vi "niUSRP EX Full Duplex (Single Device, Multi Channel)-20221205.vi"() -> ()   [LabVIEW 2021]
doc: "Continuously acquires and generates two communications signals in a synchronous manner using both channels on a two channel device."
uses:
  <instrlib>/niUSRP/niUSRP Timestamp.ctl
  <vilib>/Analysis/3filter.llb/Filter Passband Type.ctl
  <instrlib>/niUSRP/niUSRP Configure Time Start Trigger.vi
  <vilib>/Analysis/3filter.llb/Butterworth Filter (CDB).vi
  <instrlib>/niUSRP/niUSRP Fetch Rx Data (2D CDB).vi
  <vilib>/measure/maspectr.llb/FFT Power Spectrum for 1 Chan (CDB).vi
  <instrlib>/niUSRP/niUSRP Write Tx Data (2D CDB).vi
  <vilib>/measure/NI_MABase.lvlib
  <vilib>/measure/NI_MAPro.lvlib
  <vilib>/Analysis/NI_AALBase.lvlib
panel:
  out "error":i32
  in  "filter type":T1=enum."Bandpass"
  out "appended array":cdb[][](array[numeric])
  in  "low cutoff freq: fl":dbl=0.12500000000000006 format="%^.4e"
  in  "high cutoff freq: fh":dbl=0.45000000000000007 format="%^.2e"
  in  "sampling freq: fs":dbl=1.0 format="%^.2e"
  out "IQ Graph 2":dbl[][](graph)
  out "Model":string
  out "error out":errorcluster
  in  "Tab Control 2":enum32{"NI-294x/295x/X410", "NI-2900/2901"}(tab)
  in  "channel 0 carrier\n frequency [Hz]":dbl=2000000000.0 format="%#_6p"
  in  "channel 1 carrier\n frequency [Hz]":dbl=2000000000.0 format="%#_6p"
  in  "Start Trigger Time":T2={"whole seconds"=1, "fractional seconds"=0.0}
  in  "Tx Active Antenna":string="TX1"
  in  "Tab Control":T3(tab)
  out "IQ Graph":dbl[][](graph)
  out "Baseband Power Spectrum":cluster{"f0":dbl, "df":dbl, "magnitude":dbl[]}[](graph)
  in  "Stop":bool
  in  "Channel 1\nTone Amplitude":dbl=0.4 step=0.05 format="%#.6g"
  in  "Channel 1\nTone Frequency":dbl=35000.0 format="%#_6p"
  in  "Channel 0\nTone Amplitude":dbl=0.707 step=0.05 format="%#.6g"
  in  "Channel 0 \nTone Frequency":dbl=10000.0 format="%#_6p"
  out "Tx Waveform Graph":waveform(dbl)[](graph)
  in  "Waveform Size":dbl=10000.0
  in  "Rx Active Antenna":string="RX2"
  in  "Device Name":refnum<k15>="X310"
  in  "Tx Gain":dbl=1.0 format="%#_6f"
  in  "Tx IQ Rate":dbl=1000000.0 format="%#_6p"
  in  "Rx Gain":dbl=1.0 format="%#_6f"
  in  "Rx IQ Rate":dbl=1000000.0 format="%#_6p"
  # "Rx Settings"
  # "Tx Settings"
  # "For X410 use TX/RX0"
  # "Note that on the NI-2900 and NI-2901, both Rx channels share an LO and both Tx channels share an LO. However, on the NI-294x/295x devices, Rx and Tx of channel 0 share an LO and Rx and Tx of channel 1 share an LO."
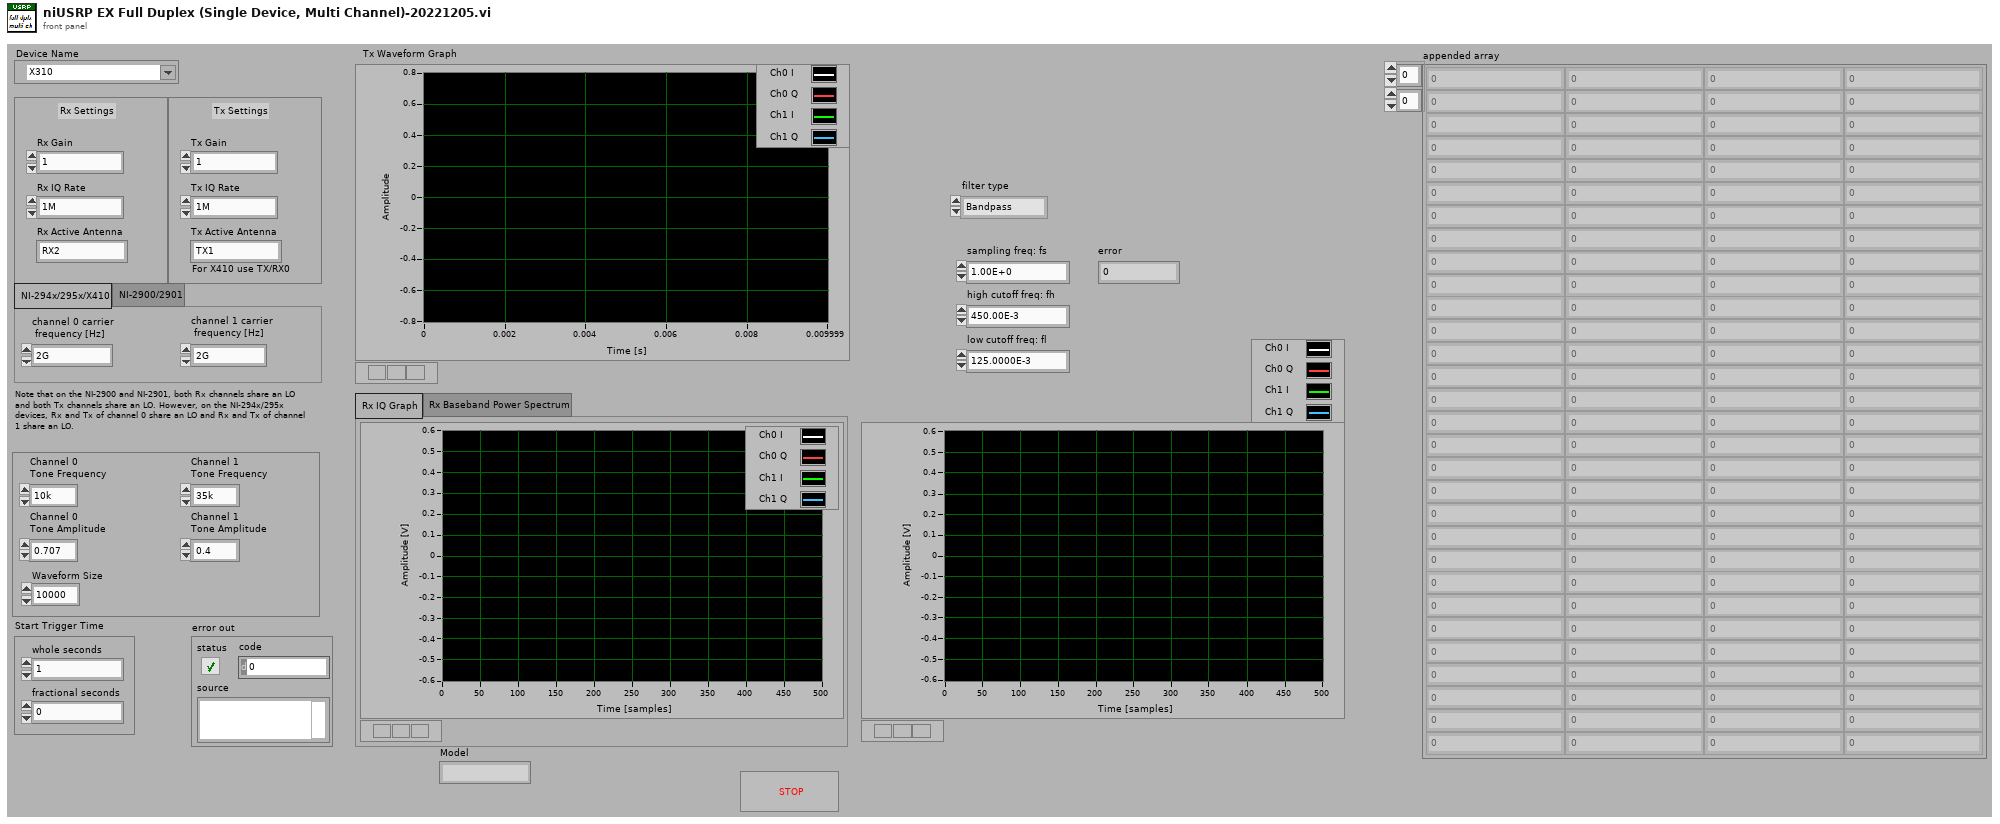
[diagram p1: front panel]
types:
  T1 = typedef "NI_AALBase.lvlib/Filter Passband Type.ctl" = enum32{"Lowpass", "Highpass", "Bandpass", "Bandstop"}
  T2 = typedef "niUSRP Timestamp.ctl" = cluster{"whole seconds":u64, "fractional seconds":dbl}
  T3 = enum32{"Rx IQ Graph", "Rx Baseband Power Spectrum"}
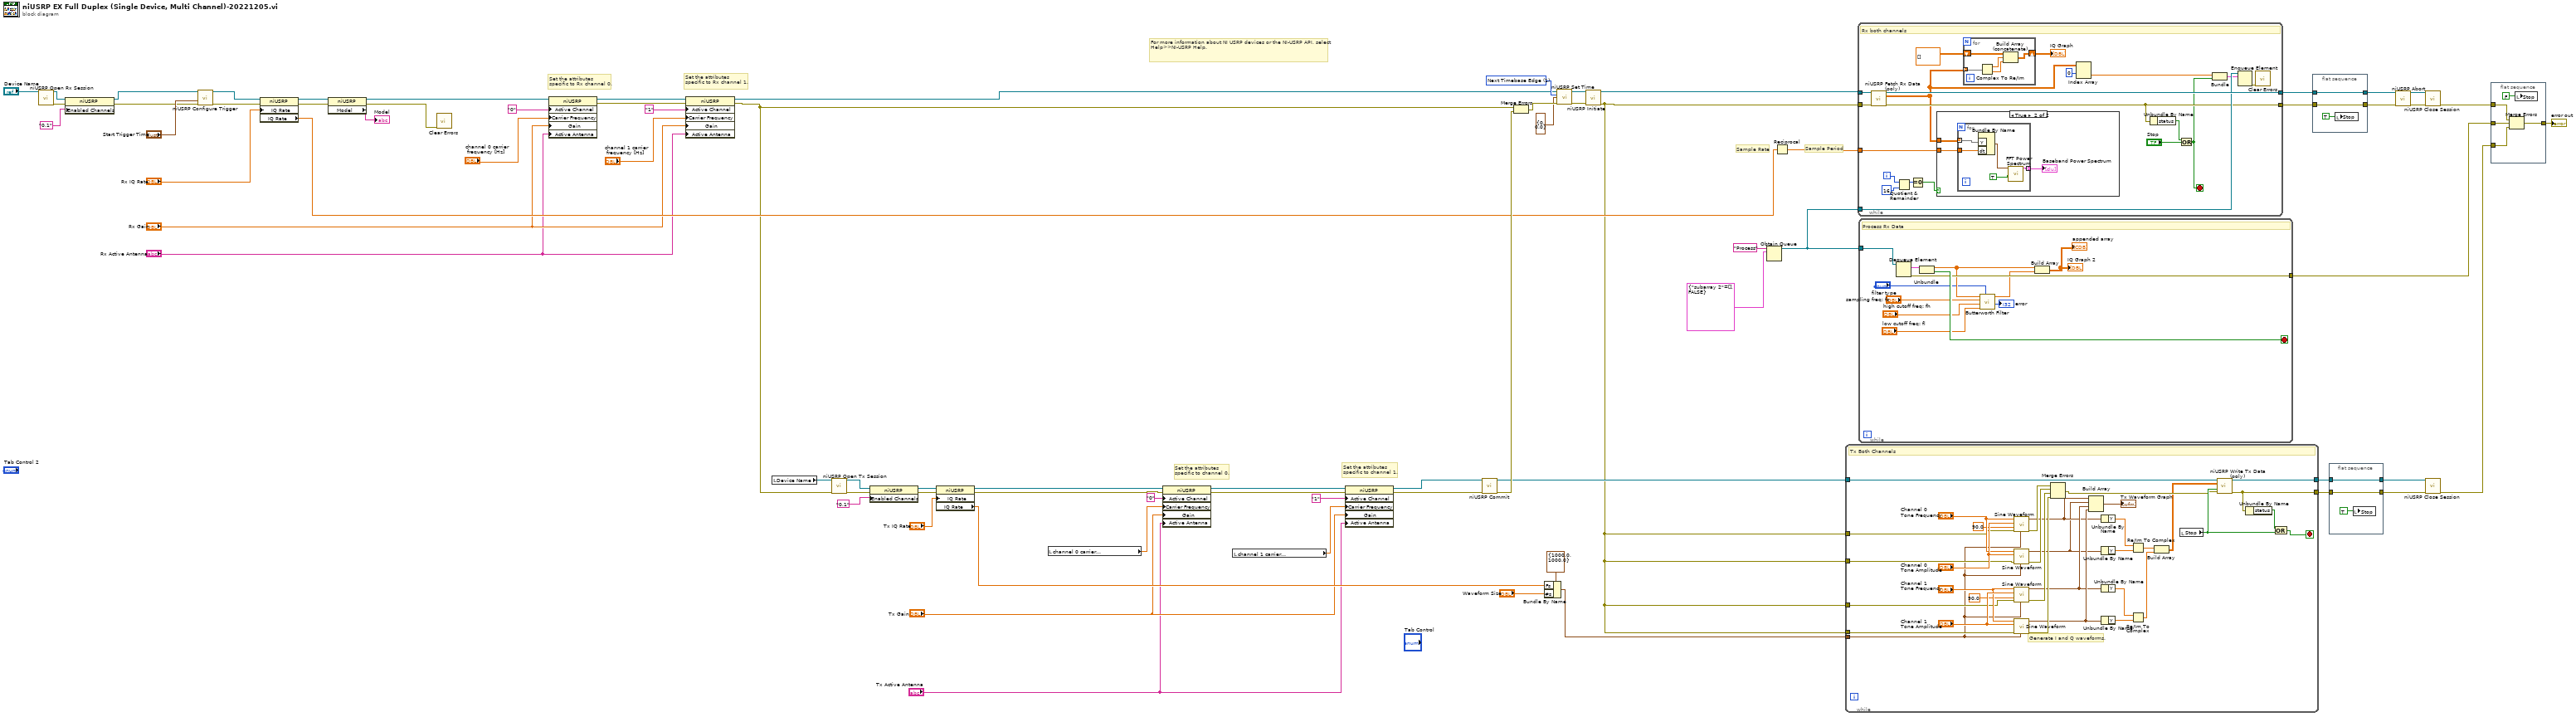
[diagram p0: block diagram]
diagram:
  w59 = 1 items=["Now", "Next Timebase Edge"] ("apply timestamp")
  # "Set the attributes \nspecific to channel 1."
  # "Set the attributes \nspecific to channel 0."
  # "Set the attributes \nspecific to Rx channel 1."
  # "Set the attributes \nspecific to Rx channel 0."
  # "Sample Rate"
  # "Sample Period"
  # "For more information about NI USRP devices or the NI-USRP API, select Help>>NI-USRP Help."
  n1 = call <instrlib>:"niUSRP Open Rx Session.vi"("device names"="Device Name") -> ("session handle out"=w58:refnum<k15>, "error out"=w57:errorcluster)  [unwired: 13 in]
  n2 = property class="niUSRP"(reference=w58, error in=w57, "Enabled Channels"="0,1" ("Configuration:Enabled Channels")) -> (reference out=w56:refnum<k15>, error out=w55:errorcluster)
  n3 = call-poly <instrlib>:"niUSRP Configure Trigger.vi"("session handle"=w56, "start trigger time"="Start Trigger Time", "error in (no error)"=w55) -> ("session handle out"=w52:refnum<k15>, "error out"=w51:errorcluster)  [unwired: 11 in]
  n4 = property class="niUSRP"(reference=w52, error in=w51, "IQ Rate"="Rx IQ Rate") -> (reference out=w47:refnum<k15>, error out=w48:errorcluster, "IQ Rate"=w49:dbl)
  n5 = property class="niUSRP"(reference=w47, error in=w48) -> (reference out=w44:refnum<k15>, error out=w5:errorcluster, "Model"=→"Model":string)
  n6 = call <vilib>:"Clear Errors.vi"("error in (no error)"=w5) -> ()  [unwired: 5 in, 2 out]
  n7 = property class="niUSRP"(reference=w44, "Active Channel"="0", "Carrier Frequency"="channel 0 carrier\n frequency [Hz]", "Gain"="Rx Gain", "Active Antenna"="Rx Active Antenna") -> (reference out=w18:refnum<k15>, error out=w17:errorcluster)  [unwired: 1 in]
  n8 = property class="niUSRP"(reference=w18, error in=w17, "Active Channel"="1", "Carrier Frequency"="channel 1 carrier\n frequency [Hz]", "Gain"="Rx Gain", "Active Antenna"="Rx Active Antenna") -> (reference out=w46:refnum<k15>, error out=w45:errorcluster)
  n9 = local read "Device Name"() -> (w70:refnum<k15>)
  n10 = call <instrlib>:"niUSRP Open Tx Session.vi"("device names"=w70, "error in (no error)"=w45) -> ("session handle out"=w54:refnum<k15>, "error out"=w53:errorcluster)  [unwired: 12 in]
  n11 = property class="niUSRP"(reference=w54, error in=w53, "Enabled Channels"="0,1" ("Configuration:Enabled Channels")) -> (reference out=w41:refnum<k15>, error out=w40:errorcluster)
  n12 = property class="niUSRP"(reference=w41, error in=w40, "IQ Rate"="Tx IQ Rate") -> (reference out=w37:refnum<k15>, error out=w38:errorcluster, "IQ Rate"=w36:dbl)
  n13 = local read "channel 0 carrier\n frequency [Hz]"() -> (w7:dbl)
  n14 = property class="niUSRP"(reference=w37, error in=w38, "Active Channel"="0", "Carrier Frequency"=w7, "Gain"="Tx Gain", "Active Antenna"="Tx Active Antenna") -> (reference out=w11:refnum<k15>, error out=w10:errorcluster)
  n15 = local read "channel 1 carrier\n frequency [Hz]"() -> (w6:dbl)
  n16 = property class="niUSRP"(reference=w11, error in=w10, "Active Channel"="1", "Carrier Frequency"=w6, "Gain"="Tx Gain", "Active Antenna"="Tx Active Antenna") -> (reference out=w34:refnum<k15>, error out=w35:errorcluster)
  n17 = call <instrlib>:"niUSRP Commit.vi"("session handle"=w34, "error in (no error)"=w35) -> ("session handle out"=w72:refnum<k15>, "error out"=w73:errorcluster)  [unwired: 12 in]
  n18 = Merge Errors(w45, w73) -> (w61:errorcluster)
  n19 = Bundle By Name(cluster=cluster{"Fs":dbl, "#s":dbl} {"Fs"=1000.0, "#s"=1000.0} ("sampling info"), "Fs"=w36, "#s"="Waveform Size") -> (w20:cluster{"Fs":dbl, "#s":dbl})
  n20 = call <instrlib>:"niUSRP Set Time.vi"("session handle"=w46, "apply timestamp"=w59, "timestamp"=T2 {"whole seconds"=0, "fractional seconds"=0.0}, "error in (no error)"=w61) -> ("session handle out"=w63:refnum<k15>, "error out"=w62:errorcluster)  [unwired: 10 in]
  n21 = call <instrlib>:"niUSRP Initiate.vi"("session handle"=w63, "error in (no error)"=w62) -> ("session handle out"=w76:refnum<k15>, "error out"=w19:errorcluster)  [unwired: 12 in]
  n22 = Obtain Queue(name (unnamed)="Process", element data type=cluster{"subarray 2":cdb[], bool} {"subarray 2"=[], FALSE}) -> (queue out=w3:refnum<queue>)  [unwired: 3 in, 2 out]
  n23 = Reciprocal(x=w49) -> (1/x=w65:dbl)
  n24 = while {
    tunnel: w72 -> [w110]
    tunnel: [w108] -> w32
    tunnel: [w106] -> w25
    tunnel: w20 -> [w81]
    tunnel: w19 -> [w85]
    tunnel: w19 -> [w84]
    tunnel: w19 -> [w82]
    tunnel: w19 -> [w80]
    stop <- w107 stop-if-true
    # "Generate I and Q waveforms."
    # "Tx Both Channels"
    n25 = call <vilib>:"Sine Waveform.vi"("sampling info"=w81, "error in (no error)"=w80, "phase"=90.0, "amplitude"="Channel 0\nTone Amplitude", "frequency"="Channel 0 \nTone Frequency") -> ("error out"=w104:errorcluster, "signal out"=w88:waveform(dbl))  [unwired: 5 in]
    n26 = call <vilib>:"Sine Waveform.vi"("sampling info"=w81, "error in (no error)"=w82, "amplitude"="Channel 0\nTone Amplitude", "frequency"="Channel 0 \nTone Frequency") -> ("error out"=w103:errorcluster, "signal out"=w87:waveform(dbl))  [unwired: 6 in]
    n27 = call <vilib>:"Sine Waveform.vi"("sampling info"=w81, "error in (no error)"=w84, "phase"=90.0, "amplitude"="Channel 1\nTone Amplitude", "frequency"="Channel 1\nTone Frequency") -> ("error out"=w102:errorcluster, "signal out"=w97:waveform(dbl))  [unwired: 5 in]
    n28 = call <vilib>:"Sine Waveform.vi"("sampling info"=w81, "error in (no error)"=w85, "amplitude"="Channel 1\nTone Amplitude", "frequency"="Channel 1\nTone Frequency") -> ("error out"=w101:errorcluster, "signal out"=w98:waveform(dbl))  [unwired: 6 in]
    n29 = Merge Errors(w104, w103, w102, w101) -> (w78:errorcluster)
    n30 = Build Array(w88, w87, w97, w98) -> (→"Tx Waveform Graph":waveform(dbl)[])
    n31 = Unbundle By Name(w88) -> ("Y"=w89:dbl[])
    n32 = Unbundle By Name(w87) -> ("Y"=w90:dbl[])
    n33 = Unbundle By Name(w97) -> ("Y"=w94:dbl[])
    n34 = Unbundle By Name(w98) -> ("Y"=w95:dbl[])
    n35 = Re/Im To Complex(1:w90, 2:w89) -> (0:w99:cdb[])
    n36 = Re/Im To Complex(1:w95, 2:w94) -> (0:w100:cdb[])
    n37 = Build Array(w99, w100) -> (w77:cdb[][])
    n38 = local read "Stop"() -> (w105:bool)
    n39 = call-poly <instrlib>:"niUSRP Write Tx Data (poly).vi"("session handle"=w110, "data"=w77, "end of data?"=w105, "error in (no error)"=w78) -> ("session handle out"=w106:refnum<k15>, "error out"=w108:errorcluster)  [unwired: 10 in]
    n40 = Unbundle By Name(w108) -> ("status"=w109:bool)
    n41 = Compound Arithmetic op=OR(w109, w105) -> (w107:bool)
  }
  n42 = while {
    tunnel: w76 -> [w130]
    tunnel: w19 -> [w129]
    tunnel: [w114] -> w30
    tunnel: [w128] -> w27
    tunnel: w65 -> [w121]
    tunnel: w3 -> [w119]
    i -> [w124]
    stop <- w113 stop-if-true
    # "Rx both channels"
    n43 = call-poly <instrlib>:"niUSRP Fetch Rx Data (poly).vi"("session handle"=w130, "error in (no error)"=w129) -> ("session handle out"=w128:refnum<k15>, "data"=w111:cdb[][], "error out"=w114:errorcluster)  [unwired: 10 in, 1 out]
    n44 = Quotient & Remainder(x=w124, y=16) -> (x-y*floor(x/y)=w127:i32)  [unwired: 1 out]
    n45 = Equal To 0?(x=w127) -> (x = 0?=w123:bool)
    n46 = case shown="True" w123 {
      tunnel: w111 -> [_ w138]
      tunnel: w121 -> [_ w137]
      frame False {
      }
      frame True {
        n47 = for {
          tunnel: w138 -> [w141] mode=indexing
          tunnel: w137 -> [w140]
          tunnel: [w139] -> w136 mode=indexing
          n48 = Bundle By Name("Y"=w141, "dt"=w140) -> (w142:waveform(cdb))  [unwired: 1 in]
          n49 = call-poly <vilib>:"FFT Power Spectrum.vi"("dB On (F)"=TRUE, "time signal"=w142) -> ("power spectrum"=w139:cluster{"f0":dbl, "df":dbl, "magnitude":dbl[]})  [unwired: 6 in, 3 out]
        }
        "Baseband Power Spectrum" <- w136
      }
    }
    n50 = for {
      tunnel: w111 -> [w135] mode=indexing
      shift-right: [w132] -> w120
      shift-left: dbl[][] [] -> [w131]
      n51 = Complex To Re/Im(x + iy=w135) -> (x=w134:dbl[], y=w133:dbl[])
      n52 = Build Array (concatenate)(w131, w134, w133) -> (w132:dbl[][])
    }
    "IQ Graph" <- w120
    n53 = Index Array(array=w111, index (row)=0) -> (element=w117:cdb[])  [unwired: 1 in]
    n54 = Unbundle By Name(w114) -> ("status"=w125:bool)
    n55 = Or(x=w125, y="Stop") -> (x .or. y?=w113:bool)
    n56 = Bundle("data"=w117, w113) -> (w116:cluster{"data":cdb[], bool})  [unwired: 1 in]
    n57 = Enqueue Element(queue=w119, element=w116) -> (error out=w118:errorcluster)  [unwired: 2 in, 2 out]
    n58 = call <vilib>:"Clear Errors.vi"("error in (no error)"=w118) -> ()  [unwired: 5 in, 2 out]
  }
  n59 = while {
    tunnel: w3 -> [w155]
    tunnel: [w152] -> w1
    stop <- w153 stop-if-true
    # "Process Rx Data"
    n60 = Dequeue Element(queue=w155) -> (element=w154:cluster{"subarray 2":cdb[], bool}, error out=w152:errorcluster)  [unwired: 2 in, 2 out]
    n61 = Unbundle(w154) -> ("subarray 2"=w151:cdb[], w153:bool)
    n62 = call-poly <vilib>:"Butterworth Filter.vi"("filter type"="filter type", "low cutoff freq: fl"="low cutoff freq: fl", "high cutoff freq: fh"="high cutoff freq: fh", "sampling freq: fs"="sampling freq: fs", "X"=w151) -> ("error"=→"error":i32, "Filtered X"=w146:cdb[])  [unwired: 3 in]
    n63 = Build Array(w151, w146) -> (→"IQ Graph 2" →"appended array":cdb[][])
  }
  n64 = flat-sequence {
    tunnel: [w157] -> w29
    tunnel: w30 -> [w157]
    tunnel: [w156] -> w28
    tunnel: w27 -> [w156]
    frame #0 {
      n65 = local write "Stop"(TRUE ("STOP")) -> ()
    }
  }
  n66 = flat-sequence {
    tunnel: [w160] -> w31
    tunnel: w32 -> [w160]
    tunnel: [w159] -> w26
    tunnel: w25 -> [w159]
    frame #0 {
      n67 = local write "Stop"(TRUE ("STOP")) -> ()
    }
  }
  n68 = call <instrlib>:"niUSRP Abort.vi"("session handle"=w28, "error in (no error)"=w29) -> ("session handle out"=w69:refnum<k15>, "error out"=w68:errorcluster)  [unwired: 12 in]
  n69 = call <instrlib>:"niUSRP Close Session.vi"("session handle"=w69, "error in (no error)"=w68) -> ("error out"=w24:errorcluster)  [unwired: 13 in]
  n70 = call <instrlib>:"niUSRP Close Session.vi"("session handle"=w26, "error in (no error)"=w31) -> ("error out"=w23:errorcluster)  [unwired: 13 in]
  n71 = flat-sequence {
    tunnel: w24 -> [w165]
    tunnel: w23 -> [w164]
    tunnel: [w163] -> w22
    tunnel: w1 -> [w162]
    frame #0 {
      n72 = Merge Errors(w165, w162, w164) -> (w163:errorcluster)
      n73 = local write "Stop"(FALSE ("STOP")) -> ()
    }
  }
  "error out" <- w22
